vi "Get_Cartesian_Command.vi"(8 "error in (no error)":errorcluster) -> (0 "error out":errorcluster, 2 "CartesianPosition":T1)   [LabVIEW 2019, in "Kinova MICO² USB.lvlib"]
uses:
  <vilib>/Utility/error.llb/Error Cluster From Error Code.vi
  <vilib>/ErrorRing/Error Ring.xnode
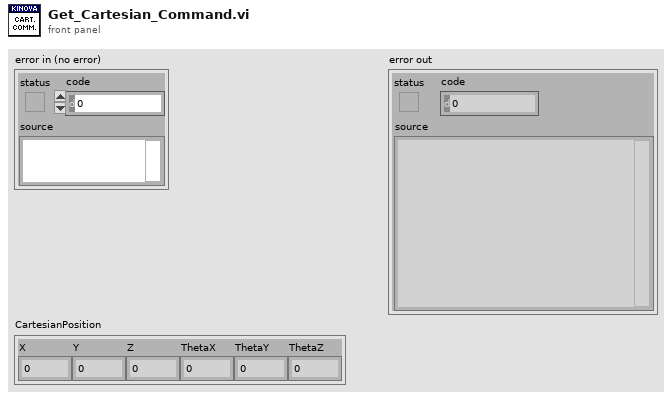
[diagram p1: front panel]
types:
  T1 = cluster{"X":sgl, "Y":sgl, "Z":sgl, "ThetaX":sgl, "ThetaY":sgl, "ThetaZ":sgl}
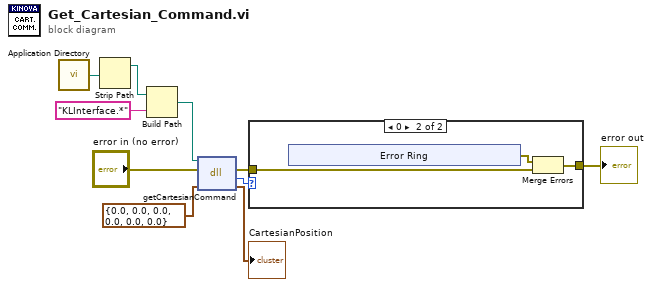
[diagram p0: block diagram]
diagram:
  n1 = call <vilib>:"Application Directory.vi"() -> ("Application Directory"=w1:path)
  n2 = Strip Path(path=w1) -> (stripped path=w7:path)  [unwired: 1 out]
  n3 = Build Path(base path=w7, name or relative path="KLInterface.*") -> (appended path=w2:path)
  n4 = dll-call lib="C:/Users/mcjssdcc/source/repos/Kinova Labview Interface/Debug/KLInterface.dll" fn="getCartesianCommand"(path in=w2, error in="error in (no error)", "point"=T1 {"X"=0.0, "Y"=0.0, "Z"=0.0, "ThetaX"=0.0, "ThetaY"=0.0, "ThetaZ"=0.0} ("CartesianPosition")) -> (error out=w9:errorcluster, "return type"=w8:i32, "point"=→"CartesianPosition":T1)  [unwired: 1 in, 1 out]
  n5 = case shown="0" w8 {
    tunnel: [w11 w13] -> w6
    tunnel: w9 -> [w11 w12]
    frame 1, Default {
    }
    frame 0 {
      n6 = xnode "Error Ring"() -> ("error out"=w14:errorcluster)
      n7 = Merge Errors(w14, w12) -> (w13:errorcluster)
    }
  }
  "error out" <- w6
